vi "Stopwatch FGV.vi"(7 "Stopwatch Action":T1, 8 "Error In":errorcluster) -> (0 "Error Out":errorcluster, 1 "Paused?":bool, 2 "Elapsed Time":dbl)   [LabVIEW 2010]
uses:
  Stopwatch Action.ctl
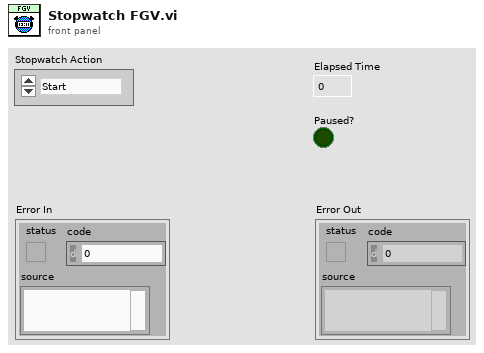
[diagram p1: front panel]
types:
  T1 = typedef "Stopwatch Action.ctl" = enum16{"Start", "Current Time", "Pause", "Reset"}
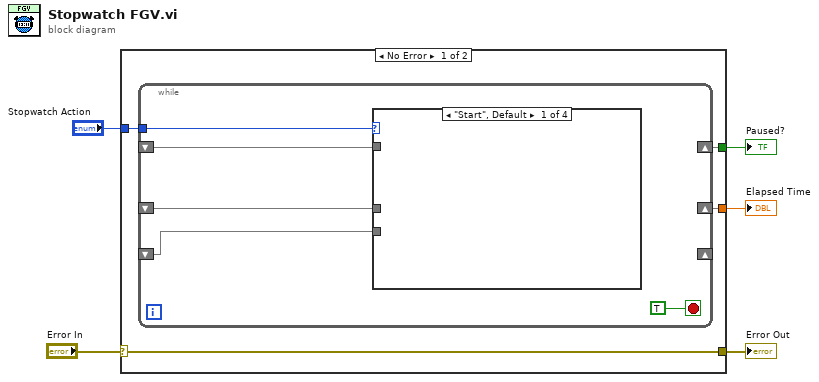
[diagram p0: block diagram]
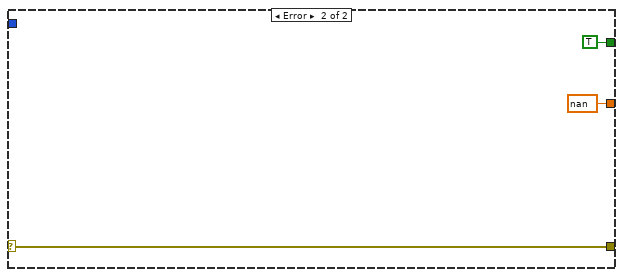
[diagram p5: hidden frame]
diagram:
  n1 = case shown="No Error" "Error In" {
    selector: "Error In" -> [w6 w17]
    tunnel: [w9 TRUE] -> w5
    tunnel: [w8 nan] -> w4
    tunnel: "Stopwatch Action" -> [w7 _]
    tunnel: [w6 w17] -> w1
    frame No Error {
      n2 = while {
        shift-right: [_] -> w8
        shift-left: _ -> [w13]
        shift-right: _ -> [_]
        shift-left: _ -> [w14]
        shift-right: [_] -> w9
        shift-left: _ -> [w11]
        tunnel: w7 -> [w10]
        stop <- TRUE stop-if-true
        n3 = case shown="\"Start\", Default" w10 {
          tunnel: w13 -> [_ _ _ _]
          tunnel: w11 -> [_ _ _ _]
          tunnel: w14 -> [_ _ _ _]
          frame "Start", Default {
          }
          frame "Pause" {
          }
          frame "Reset" {
          }
          frame "Current Time" {
          }
        }
      }
    }
    frame Error {
    }
  }
  "Paused?" <- w5
  "Elapsed Time" <- w4
  "Error Out" <- w1
